vi "NI VeriStand - Get Model List.vi"(7 "Target":string, 8 "error in (no error)":errorcluster, 11 "ModelManager in":T1) -> (0 "error out":errorcluster, 2 "Models":string[](array[string]), 3 "ModelManager out":T1)   [LabVIEW 2020, in "NI_VS ModelManager ExecutionAPI.lvlib"]
doc: "Returns a list of all the models running on the target."
uses:
  <vilib>/NI VeriStand/Execution/ModelManager/NI_VS ModelManager ExecutionAPI.lvlib
  <vilib>/NI VeriStand/Execution/ModelManager/ModelManagerAPI.ctl
  NationalInstruments.VeriStand.ClientAPI
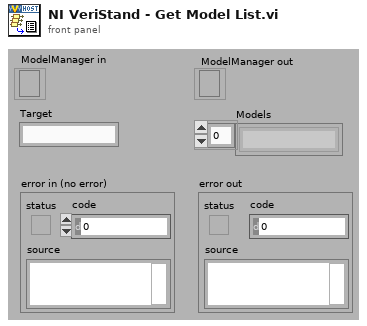
[diagram p1: front panel]
types:
  T1 = typedef "NI_VS ModelManager ExecutionAPI.lvlib/ModelManagerAPI.ctl" = refnum<k24>
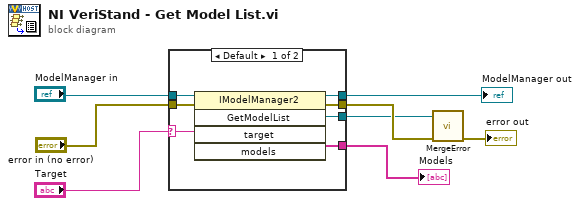
[diagram p0: block diagram]
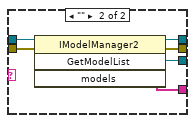
[diagram p2: hidden frame]
diagram:
  n1 = case shown="Default" "Target" {
    selector: "Target" -> [w9 _]
    tunnel: "ModelManager in" -> [w15 w21]
    tunnel: [w14 w20] -> w7
    tunnel: [w13 w19] -> w6
    tunnel: [w12 w18] -> w5
    tunnel: "error in (no error)" -> [w11 w17]
    tunnel: [w10 w16] -> w2
    frame Default {
      n2 = invoke class="IModelManager2" method="GetModelList"(reference=w15, error in=w11, "target"=w9) -> (reference out=w14:T1, error out=w13:errorcluster, "GetModelList"=w12:refnum<k24>, "models"=w10:string[])  [unwired: 2 in, 1 out]
    }
    frame "" {
      n3 = invoke class="IModelManager2" method="GetModelList"(reference=w21, error in=w17) -> (reference out=w20:T1, error out=w19:errorcluster, "GetModelList"=w18:refnum<k24>, "models"=w16:string[])  [unwired: 2 in]
    }
  }
  "ModelManager out" <- w7
  "Models" <- w2
  n4 = call <vilib>:"MergeError.vi"("error in (no error)"=w6, "Error"=w5) -> ("error out"=→"error out":errorcluster)  [unwired: 9 out]
